vi "send_email.vi"(8 "error in (no error)":errorcluster, 10 "attachments array in":path[](array[path]), 11 "ErrorController in":refnum<class "ErrorController.lvclass">) -> (0 "error out":errorcluster, 2 "attachments array out":path[](array[path]), 3 "ErrorController out":refnum<class "ErrorController.lvclass">)   [LabVIEW 2010, in "ErrorController.lvclass"]
uses:
  ErrorController.lvclass
  ErrorController.lvclass/ErrorController.ctl
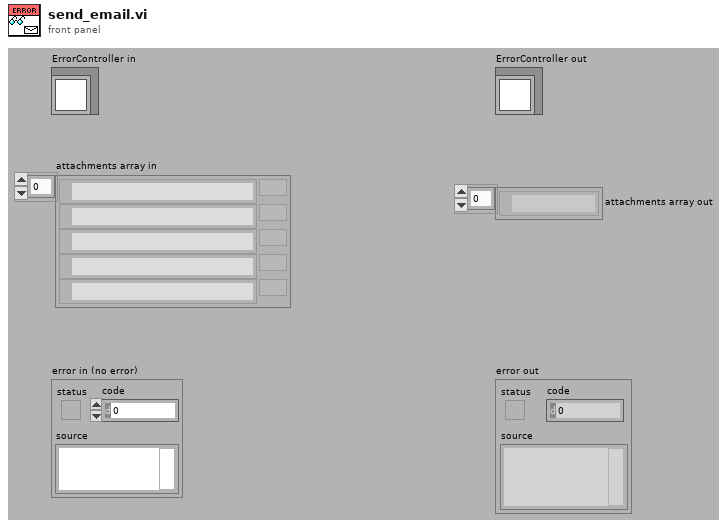
[diagram p1: front panel]
types:
  T1 = enum16{"open", "replace", "create", "open or create", "replace or create", "replace or create with confirmation"}
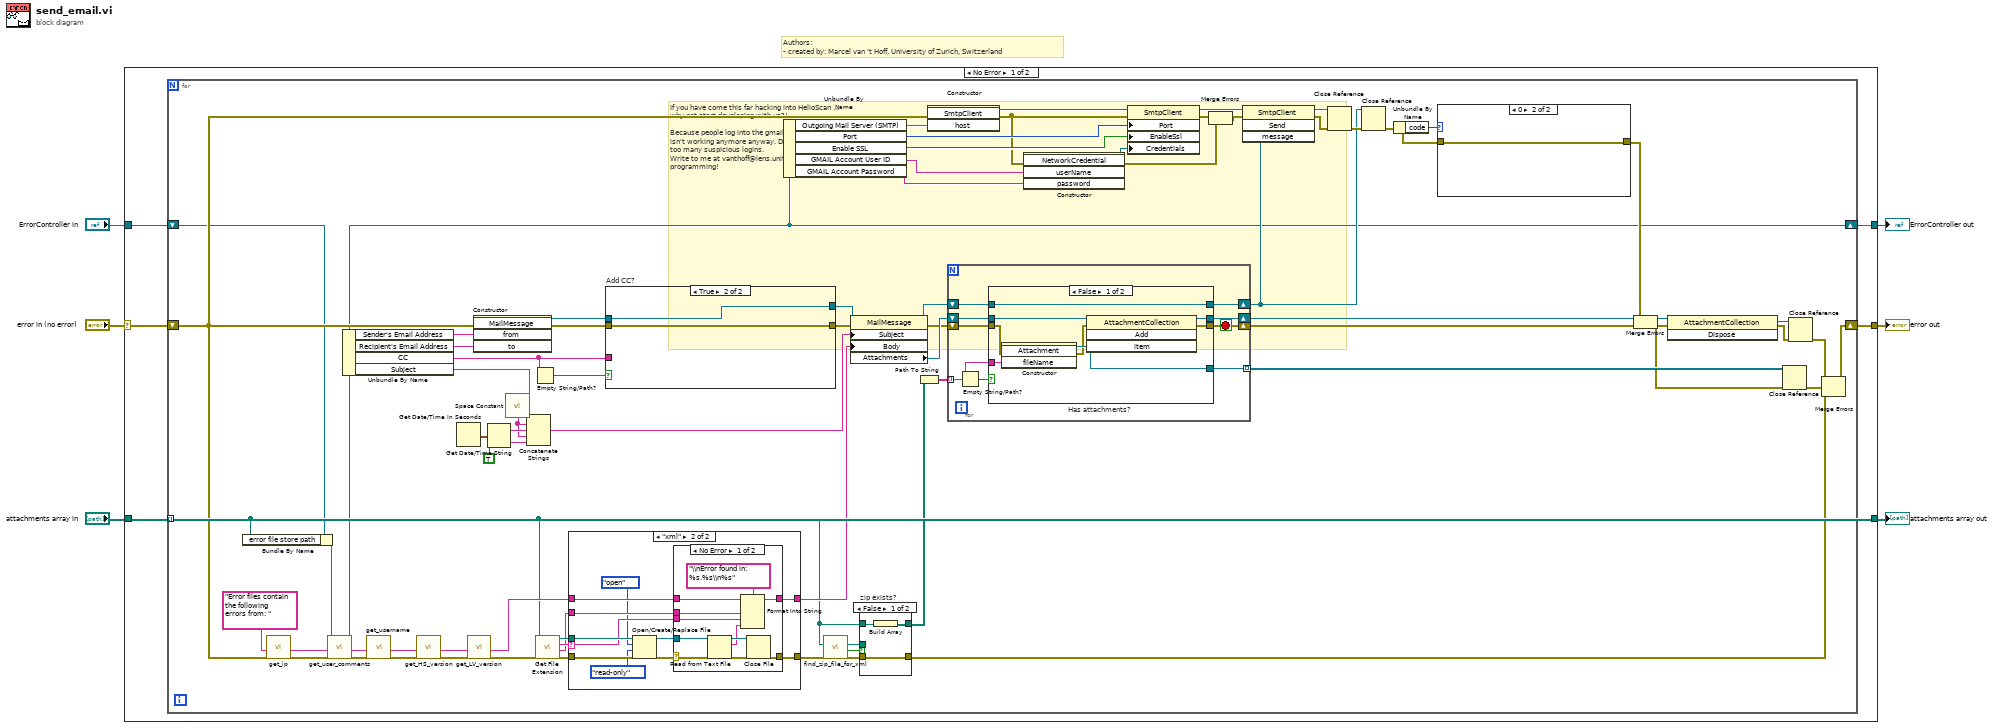
[diagram p0: block diagram]
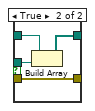
[diagram p2: hidden frame]
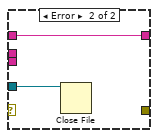
[diagram p4: hidden frame]
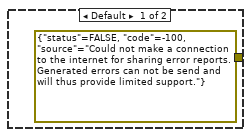
[diagram p5: hidden frame]
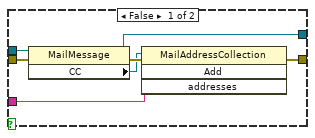
[diagram p7: hidden frame]
diagram:
  # "Authors: \n- created by: Marcel van 't Hoff, University of Zurich, Switzerland"
  n1 = case shown="No Error" "error in (no error)" {
    selector: "error in (no error)" -> [w10 w151]
    tunnel: "ErrorController in" -> [w11 w152]
    tunnel: [w7 w152] -> w4
    tunnel: [w8 w151] -> w3
    tunnel: "attachments array in" -> [w9 w150]
    tunnel: [w9 w150] -> w1
    frame No Error {
      n2 = for {
        tunnel: w9 -> [w16] mode=indexing
        shift-right: [w26] -> w8
        shift-left: w10 -> [w85]
        shift-right: [w12] -> w7
        shift-left: w11 -> [w25]
        # "If you have come this far hacking into HelioScan ... \nwhy not start developing with us?! \n\nBecause people log into the gmail account, the password\nisn't working anymore anyway. Don't even try. We've had\ntoo many suspicious logins.\nWrite to me at vanthoff@lens.unifi.it to get you started with\nprogramming!"
        n3 = Bundle By Name(cluster=w25, "error file store path"=w16) -> (w24:refnum<class "ErrorController.lvclass">)
        n4 = call "get_ip.vi"("error in (no error)"=w85, "string in"="Error files contain the following errors from: ") -> ("error out"=w30:errorcluster, "edited string out"=w28:string)  [unwired: 7 in, 1 out]
        n5 = call-dynamic "get_user_comments.vi"("error in (no error)"=w30, "string in"=w28, "ErrorController in"=w24) -> ("error out"=w29:errorcluster, "string out"=w27:string, "ErrorController out"=w12:refnum<class "ErrorController.lvclass">)  [unwired: 5 in, 1 out]
        n6 = Unbundle By Name(w12) -> ("Sender's Email Address"=w42:string, "Recipient's Email Address"=w73:string, "CC"=w56:string, "Subject"=w53:string)
        n7 = call "get_username.vi"("error in (no error)"=w29, "string in"=w27) -> ("error out"=w39:errorcluster, "edited string out"=w38:string)  [unwired: 8 in]
        n8 = call "get_HS_version.vi"("error in (no error)"=w39, "string in"=w38) -> ("error out"=w37:errorcluster, "version number edited string out"=w36:string)  [unwired: 7 in, 1 out]
        n9 = Get Date/Time In Seconds() -> (seconds since 1Jan1904=w59:timestamp)
        n10 = call "get_LV_version.vi"("error in (no error)"=w37, "string in"=w36) -> ("error out"=w34:errorcluster, "edited string out"=w35:string)  [unwired: 8 in]
        n11 = constructor class="MailMessage"(error in=w85, "from"=w42, "to"=w73) -> (reference out=w81:refnum<k24>, error out=w80:errorcluster)  [unwired: 2 in, 3 out]
        n12 = Get Date/Time String(seconds (now)=w59, want seconds? (F)=TRUE) -> (date string=w57:string, time string=w52:string)  [unwired: 1 in]
        n13 = call <vilib>:"Space Constant.vi"() -> ("String"=w51:string)
        n14 = Concatenate Strings(w53, w51, w57, w51, w52) -> (w54:string)
        n15 = Empty String/Path?(string/path=w56) -> (empty?=w55:bool)
        n16 = call <vilib>:"Get File Extension.vi"("error in (no error)"=w34, "file"=w16) -> ("error out"=w22:errorcluster, "filename without extension"=w20:string, "lowercase file extension"=w23:string, "dup file"=w21:path)  [unwired: 6 in]
        n17 = case shown="\"xml\"" w23 {
          selector: w23 -> [_ w99]
          tunnel: w22 -> [w93 w104]
          tunnel: w21 -> [_ w105]
          tunnel: [w93 w102] -> w19
          tunnel: [w94 w100] -> w40
          tunnel: w35 -> [w94 w101]
          tunnel: w20 -> [_ w98]
          frame Default {
          }
          frame "xml" {
            n18 = Open/Create/Replace File(file path (use dialog)=w105, error in=w104, operation (0:open)=T1."open", access (0:read/write)=enum16{"read/write", "read-only", "write-only"}."read-only") -> (refnum out=w103:refnum<file>, error out=w95:errorcluster)  [unwired: 2 in, 1 out]
            n19 = case shown="No Error" w95 {
              selector: w95 -> [w106 _]
              tunnel: w103 -> [w115 w117]
              tunnel: [w113 _] -> w102
              tunnel: w101 -> [w111 w118]
              tunnel: [w110 w118] -> w100
              tunnel: w99 -> [w109 _]
              tunnel: w98 -> [w107 _]
              frame No Error {
                n20 = Read from Text File(file (use dialog)=w115, error in=w106) -> (refnum out=w114:refnum<file>, text=w108:string, error out=w116:errorcluster)  [unwired: 2 in, 1 out]
                n21 = Format Into String(format string="\\nError found in: %s.%s\\n%s", initial string=w111, w107, w109, w108) -> (resulting string=w110:string)  [unwired: 1 in, 1 out]
                n22 = Close File(refnum=w114, error in=w116) -> (error out=w113:errorcluster)  [unwired: 1 out]
              }
              frame Error {
                n23 = Close File(refnum=w117) -> ()  [unwired: 1 in, 2 out]
              }
            }
          }
        }
        n24 = case "Add CC?" shown="True" w55 {
          tunnel: w56 -> [w145 _]
          tunnel: w81 -> [w144 w149]
          tunnel: w80 -> [w143 w148]
          tunnel: [w142 w149] -> w79
          tunnel: [w141 w148] -> w78
          frame False {
            n25 = property class="MailMessage"(reference=w144, error in=w143) -> (reference out=w142:refnum<k24>, error out=w147:errorcluster, "CC"=w146:refnum<k24>)
            n26 = invoke class="MailAddressCollection" method="Add"(reference=w146, error in=w147, "addresses"=w145) -> (error out=w141:errorcluster)  [unwired: 1 in, 3 out]
          }
          frame True {
          }
        }
        n27 = Unbundle By Name(w12) -> ("Outgoing Mail Server (SMTP)"=w72:string, "Port"=w71:i32, "Enable SSL"=w47:bool, "GMAIL Account User ID"=w69:string, "GMAIL Account Password"=w70:string)
        n28 = call "find_zip_file_for_xml.vi"("error in (no error)"=w19, "xml file in"=w16) -> ("error out"=w15:errorcluster, "file or folder exists?"=w18:bool, "new zip file out"=w17:path)  [unwired: 7 in]
        n29 = property class="MailMessage"(reference=w79, error in=w78, "Subject"=w54, "Body"=w40) -> (reference out=w48:refnum<k24>, error out=w49:errorcluster, "Attachments"=w50:refnum<k24>)
        n30 = case "zip exists?" shown="False" w18 {
          tunnel: w17 -> [_ w92]
          tunnel: w16 -> [w87 w91]
          tunnel: [w88 w90] -> w14
          tunnel: w15 -> [w88 w90]
          tunnel: [w86 w89] -> w13
          frame False {
            n31 = Build Array(w87) -> (w86:path[])
          }
          frame True {
            n32 = Build Array(w91, w92) -> (w89:path[])
          }
        }
        n33 = Path To String(path=w13) -> (string=w65:string[])
        n34 = constructor class="SmtpClient"(error in=w85, "host"=w72) -> (reference out=w82:refnum<k24>, error out=w43:errorcluster)  [unwired: 2 in, 2 out]
        n35 = for {
          tunnel: [w129] -> w84 mode=indexing
          tunnel: w65 -> [w121] mode=indexing
          shift-right: [w127] -> w74
          shift-left: w48 -> [w126]
          shift-right: [w123] -> w66
          shift-left: w49 -> [w124]
          shift-right: [w128] -> w60
          shift-left: w50 -> [w125]
          stop <- w123 stop-if-true
          n36 = Empty String/Path?(string/path=w121) -> (empty?=w122:bool)
          n37 = case "Has attachments?" shown="False" w122 {
            tunnel: w126 -> [w133 w140]
            tunnel: [w133 w140] -> w127
            tunnel: w121 -> [w137 _]
            tunnel: [w136 _] -> w129
            tunnel: w124 -> [w130 w139]
            tunnel: [w135 w139] -> w123
            tunnel: [w134 w138] -> w128
            tunnel: w125 -> [w132 w138]
            frame False {
              n38 = constructor class="Attachment"(error in=w130, "fileName"=w137) -> (reference out=w136:refnum<k24>, error out=w131:errorcluster)  [unwired: 2 in, 2 out]
              n39 = invoke class="AttachmentCollection" method="Add"(reference=w132, error in=w131, "item"=w136) -> (reference out=w134:refnum<k24>, error out=w135:errorcluster)  [unwired: 1 in, 2 out]
            }
            frame True {
            }
          }
        }
        n40 = constructor class="NetworkCredential"(error in=w43, "userName"=w69, "password"=w70) -> (reference out=w46:refnum<k24>, error out=w68:errorcluster)  [unwired: 2 in, 3 out]
        n41 = property class="SmtpClient"(reference=w82, error in=w43, "Port"=w71, "EnableSsl"=w47, "Credentials"=w46) -> (reference out=w44:refnum<k24>, error out=w45:errorcluster)
        n42 = Merge Errors(w45, w68) -> (w67:errorcluster)
        n43 = invoke class="SmtpClient" method="Send"(reference=w44, error in=w67, "message"=w74) -> (reference out=w77:refnum<k24>, error out=w76:errorcluster)  [unwired: 1 in, 2 out]
        n44 = Close Reference(reference=w77, error in (no error)=w76) -> (error out=w75:errorcluster)
        n45 = Close Reference(reference=w74, error in (no error)=w75) -> (error out=w32:errorcluster)
        n46 = Unbundle By Name(w32) -> ("code"=w33:i32)
        n47 = case shown="0" w33 {
          tunnel: w32 -> [_ w120]
          tunnel: [errorcluster {"status"=FALSE, "code"=-100, "source"="Could not make a connection to the internet for sharing error reports. Generated errors can not be send and will thus provide limited support."} ("error out") w120] -> w31
          frame Default {
          }
          frame 0 {
          }
        }
        n48 = Merge Errors(w31, w66) -> (w63:errorcluster)
        n49 = invoke class="AttachmentCollection" method="Dispose"(reference=w60, error in=w63) -> (reference out=w64:refnum<k24>, error out=w62:errorcluster)  [unwired: 1 in, 1 out]
        n50 = Close Reference(reference=w84, error in (no error)=w63) -> (error out=w61:errorcluster)
        n51 = Close Reference(reference=w64, error in (no error)=w62) -> (error out=w83:errorcluster)
        n52 = Merge Errors(w83, w61, w14) -> (w26:errorcluster)
      }
    }
    frame Error {
    }
  }
  "error out" <- w3
  "ErrorController out" <- w4
  "attachments array out" <- w1
